vi "Simulator_Core.vi"(6 "NotifierReff":T1, 10 "disp_k":dbl=80.0, 11 "dt":dbl=1.0) -> ()   [LabVIEW 2013]
doc: "Simulator Core does a single time-step update (by dt), takes in only main position, jib position, and rudder position, and dt, (everything else is purely done by shift register and updates within the simulator), and outputs the new state variables and environmental conditions. Serves as the \"MODEL\" component of a model-view-controller simulation.\n\nSimulates based on ratios between expected behavior and modifying conditions rather than attempting and then kludging a force model. See the accompanying document for expanation of modeling decisions."
uses:
  cRIO_Code/Data/TypeDefs/Notifiers.ctl
  cRIO_Code/Data/TypeDefs/UTM Location.ctl
  cRIO_Code/Data/TypeDefs/Sail Set Suggestions.ctl
  cRIO_Code/Data/TypeDefs/Rudder Set Suggestions.ctl
  cRIO_Code/Data/TypeDefs/OverrideInformation.ctl
  cRIO_Code/Data/TypeDefs/OverrideMode.ctl
  cRIO_Code/Data/TypeDefs/MotorSetup.ctl
  cRIO_Code/Data/TypeDefs/DynamixelSetupInfo.ctl
  cRIO_Code/Data/TypeDefs/AirmarStatus.ctl
  cRIO_Code/Data/TypeDefs/HardwareOnline.ctl
  cRIO_Code/Data/TypeDefs/DynamixelCycleTracker.ctl
  cRIO_Code/Data/TypeDefs/RC Input Values.ctl
  cRIO_Code/Logic/Classes/Missions/GenericMission/GenericMission.lvclass
  cRIO_Code/Logic/Classes/Waypoint/Waypoint.lvclass
panel:
  out "rel_wind":dbl
  out "rel_wind_comp":dbl
  out "angular_drag":dbl
  out "Ts":dbl
  out "Tr":dbl
  out "RobotSp":dbl
  out "Vmax":dbl
  out "Vtmax":dbl
  out "SimLoopCounter":i32
  out "RelWindAngle":dbl
  out "JibP":dbl
  out "MainP":dbl
  out "WindSpeed":dbl
  out "AbsWindDirection":dbl(knob)
  out "RobotH":dbl(knob)
  out "PosY":dbl(graph)
  out "PosX":dbl(graph)
  out "VelY":dbl(graph)
  out "VelX":dbl(graph)
  out "Angular Velocity":dbl(graph)
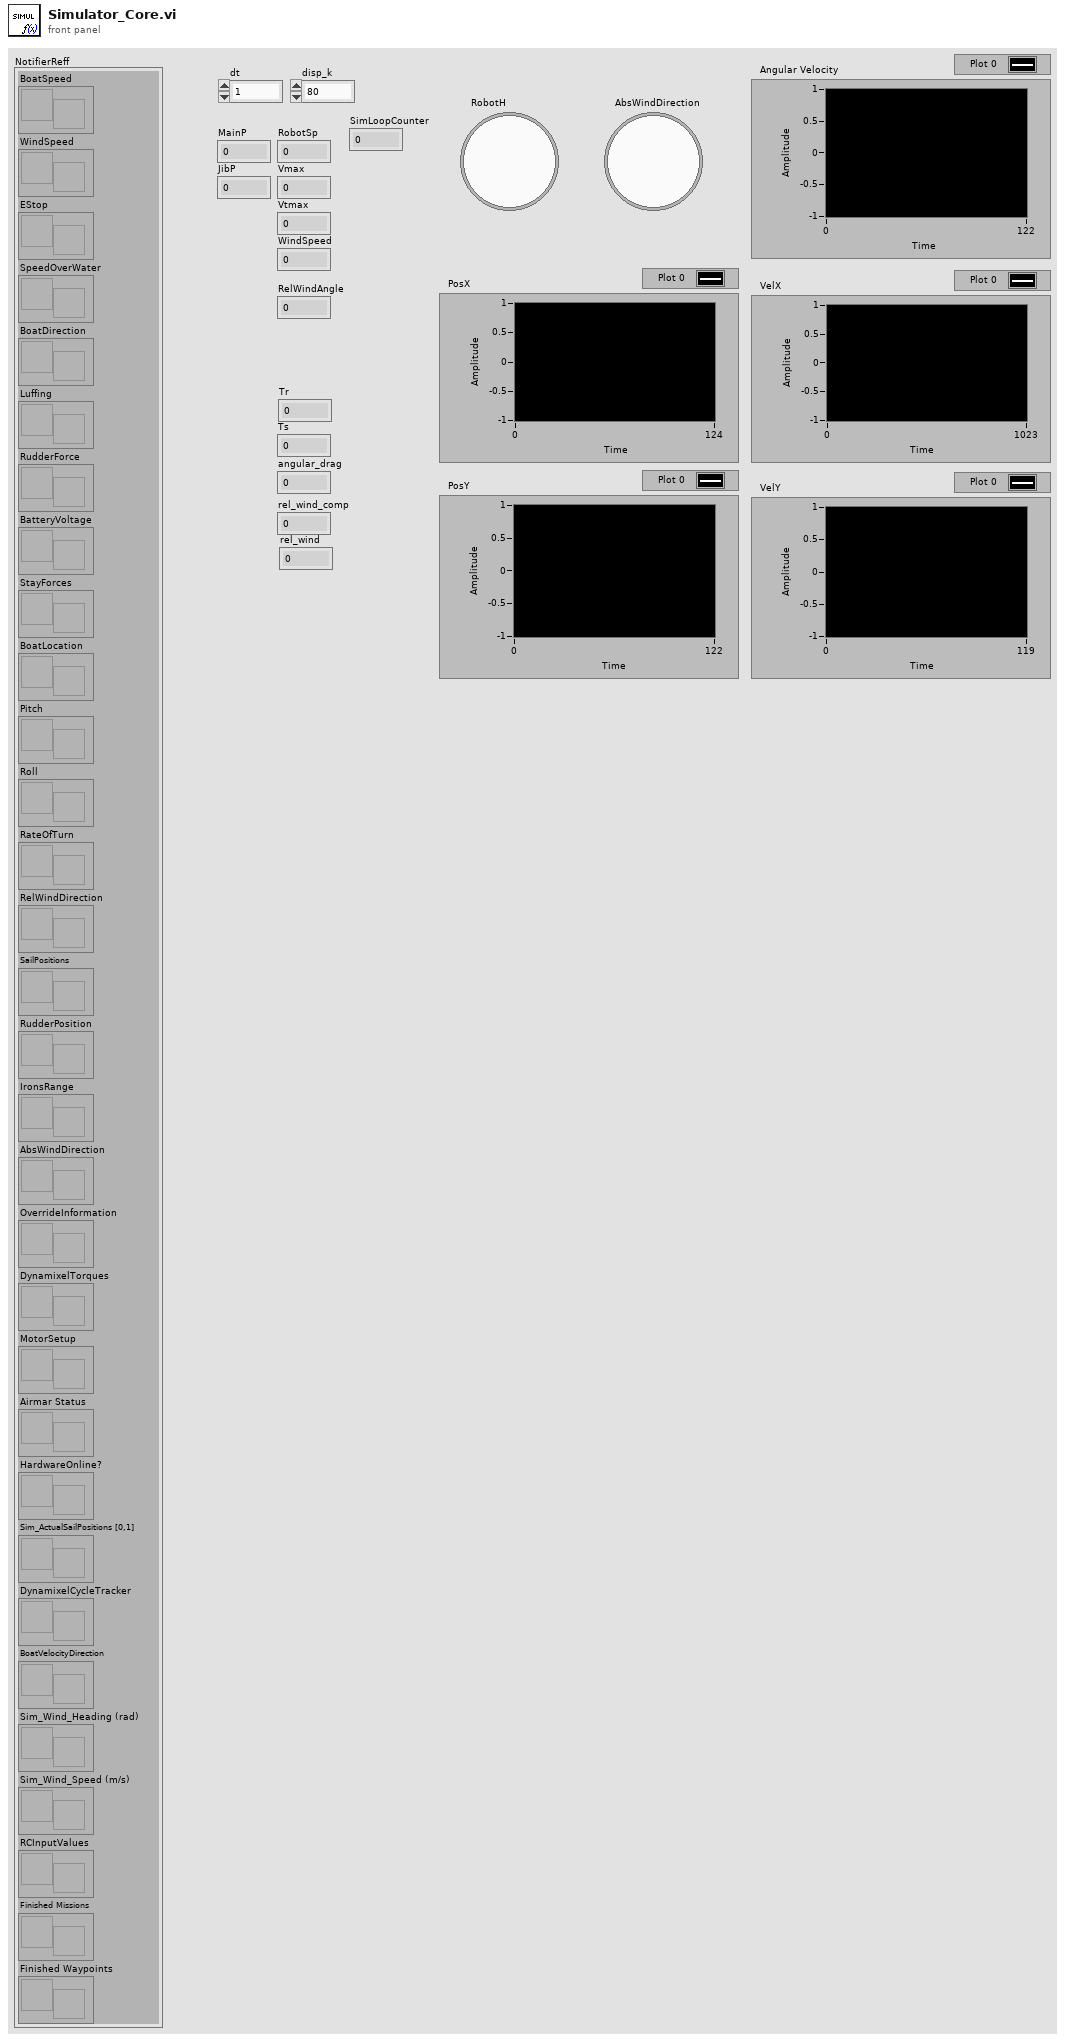
[diagram p1: front panel]
types:
  T1 = typedef "Notifiers.ctl" = cluster{"BoatSpeed":refnum<notifier>, "WindSpeed":refnum<notifier>, "EStop":refnum<notifier>, "SpeedOverWater":refnum<notifier>, "BoatDirection":refnum<notifier>, "Luffing":refnum<notifier>, "RudderForce":refnum<notifier>, "BatteryVoltage":refnum<notifier>, "StayForces":refnum<notifier>, "BoatLocation":refnum<notifier>, "Pitch":refnum<notifier>, "Roll":refnum<notifier>, "RateOfTurn":refnum<notifier>, "RelWindDirection":refnum<notifier>, "SailPositions":refnum<notifier>, "RudderPosition":refnum<notifier>, "IronsRange":refnum<notifier>, "AbsWindDirection":refnum<notifier>, "OverrideInformation":refnum<notifier>, "DynamixelTorques":refnum<notifier>, "MotorSetup":refnum<notifier>, "Airmar Status":refnum<notifier>, "HardwareOnline?":refnum<notifier>, "Sim_ActualSailPositions [0,1]":refnum<notifier>, "DynamixelCycleTracker":refnum<notifier>, "BoatVelocityDirection":refnum<notifier>, "Sim_Wind_Heading (rad)":refnum<notifier>, "Sim_Wind_Speed (m/s)":refnum<notifier>, "RCInputValues":refnum<notifier>, "Finished Missions":refnum<notifier>, "Finished Waypoints":refnum<notifier>}
  T2 = typedef "UTM Location.ctl" = cluster{"UTM Zone":dbl, "Hemisphere":enum16{"North", "South"}, "East":dbl, "North":dbl}
  T3 = typedef "Rudder Set Suggestions.ctl" = dbl
  T4 = typedef "Sail Set Suggestions.ctl" = cluster{"MainSailSuggestion":dbl, "JibSailSuggestion":dbl}
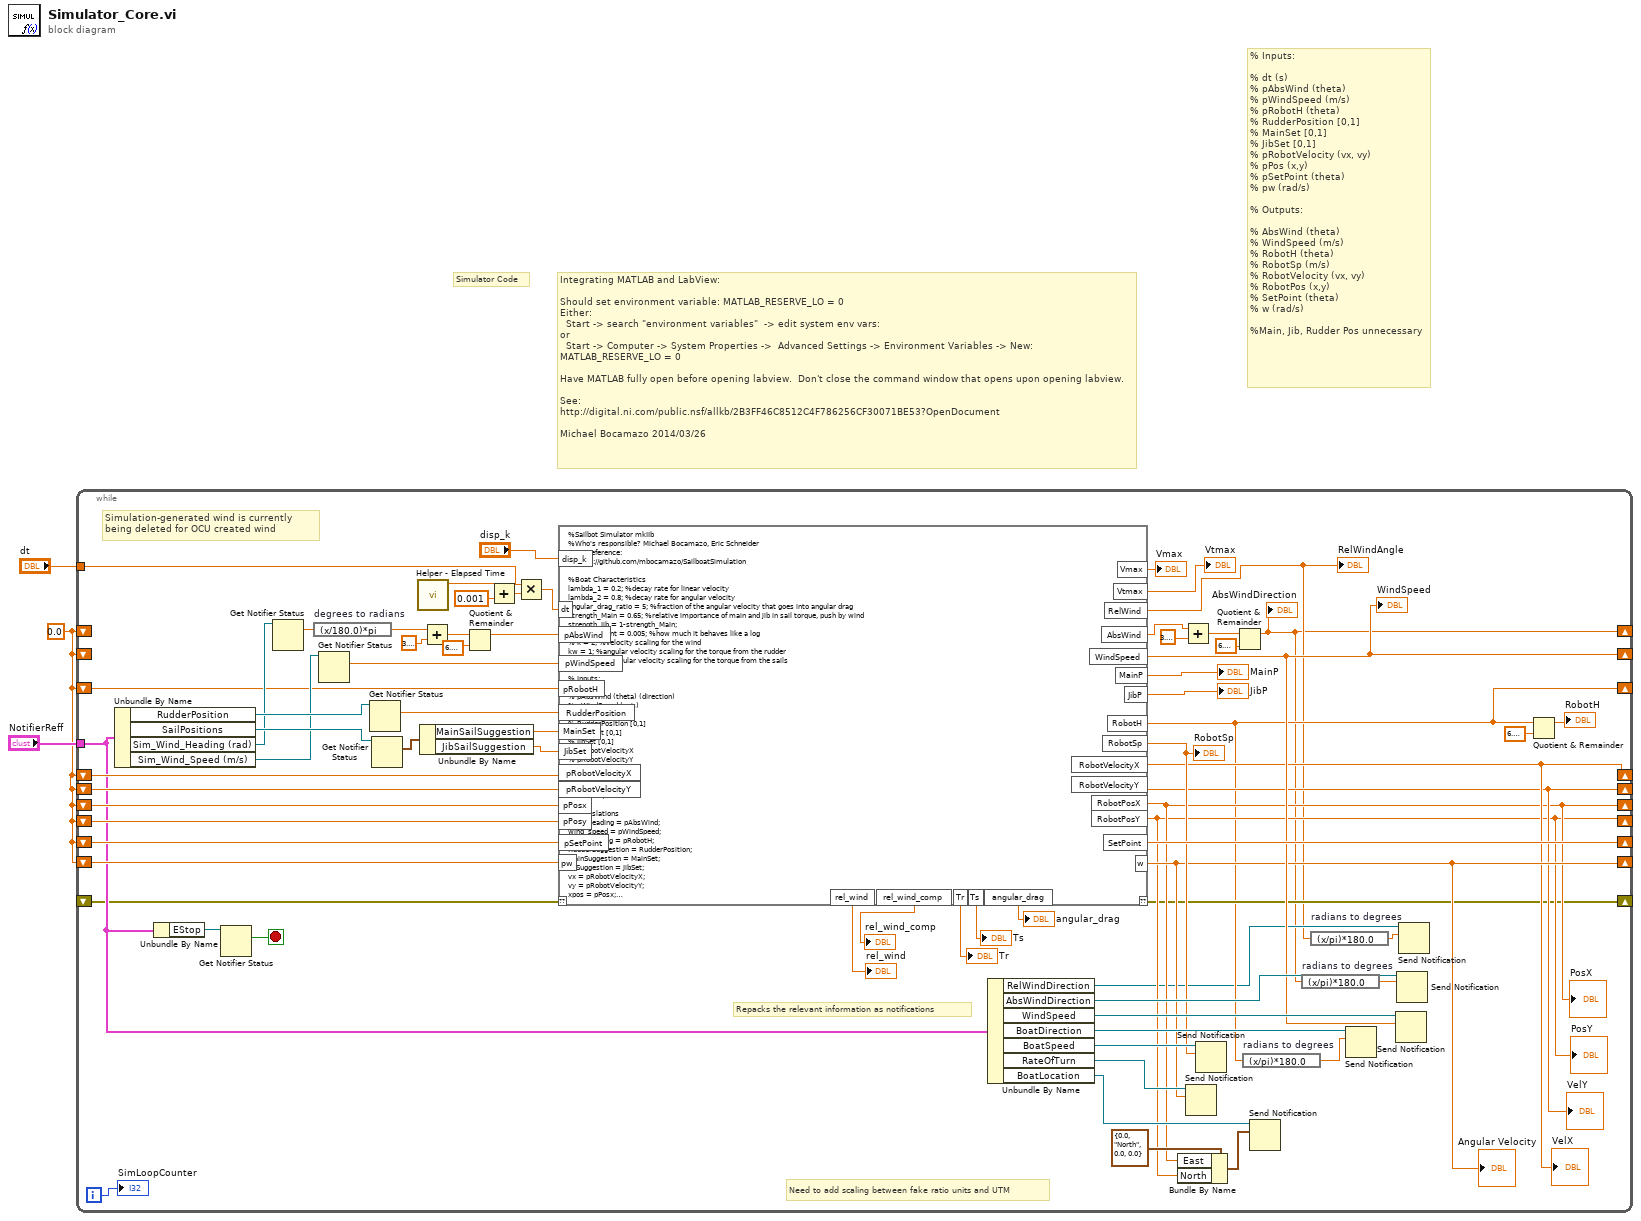
[diagram p0: block diagram]
diagram:
  w1 = 0.0
  # "% Inputs:\n\n% dt (s)\n% pAbsWind (theta)\n% pWindSpeed (m/s)\n% pRobotH (theta)\n% RudderPosition [0,1]\n% MainSet [0,1]\n% JibSet [0,1]\n% pRobotVelocity (vx, vy)\n% pPos (x,y)\n% pSetPoint (theta)\n% pw (rad/s)\n\n% Outputs:\n\n% AbsWind (theta)\n% WindSpeed (m/s)\n% RobotH (theta)\n% RobotSp (m/s)\n% RobotVelocity (vx, vy)\n% RobotPos (x,y)\n% SetPoint (theta)\n% w (rad/s)\n\n%Main, Jib, Rudder Pos unnecessary"
  # "Integrating MATLAB and LabView:\n\nShould set environment variable: MATLAB_RESERVE_LO = 0\nEither:\n  Start -> search \"environment variables\"  -> edit system env vars:\nor\n  Start -> Computer -> System Properties ->  Advanced Settings -> Environment Variables -> New:\nMATLAB_RESERVE_LO = 0 \n\nHave MATLAB fully open before opening labview.  Don't close the command window that opens upon opening labview.   \n\nSee:\nhttp://digital.ni.com/public.nsf/allkb/2B3FF46C8512C4F786256CF30071BE53?OpenDocument\n\nMichael Bocamazo 2014/03/26"
  # "Simulator Code"
  n1 = while {
    shift-right: [w54] -> _
    shift-left: w1 -> [w75]
    shift-right: [w74] -> _
    shift-left: w1 -> [w73]
    shift-right: [w51] -> _
    shift-left: w1 -> [w58]
    shift-right: [w12] -> _
    shift-left: w1 -> [_]
    shift-right: [w67] -> _
    shift-left: w1 -> [_]
    shift-right: [w33] -> _
    shift-left: w1 -> [w11]
    shift-right: [w52] -> _
    shift-left: w1 -> [w55]
    tunnel: "dt" -> [w10]
    tunnel: "NotifierReff" -> [w49]
    shift-right: [w50] -> _
    shift-left: w1 -> [w57]
    shift-right: [w53] -> _
    shift-left: w1 -> [w56]
    shift-right: [w44] -> _
    shift-left: _ -> [w43]
    i -> [w37]
    stop <- w47 stop-if-true
    # "Simulation-generated wind is currently being deleted for OCU created wind"
    # "Need to add scaling between fake ratio units and UTM"
    # "Repacks the relevant information as notifications"
    n2 = Unbundle By Name(w49) -> ("RudderPosition"=w72:refnum<notifier>, "SailPositions"=w70:refnum<notifier>, "Sim_Wind_Heading (rad)"=w31:refnum<notifier>, "Sim_Wind_Speed (m/s)"=w30:refnum<notifier>)
    n3 = Unbundle By Name(w49) -> ("EStop"=w48:refnum<notifier>)
    n4 = Get Notifier Status(notifier=w48) -> (current notification=w47:bool)  [unwired: 1 in, 4 out]
    n5 = Get Notifier Status(notifier=w31) -> (current notification=w23:dbl)  [unwired: 1 in, 4 out]
    n6 = expression code="(x/180.0)*pi" "degrees to radians"(w23) -> (w22:dbl)
    n7 = Get Notifier Status(notifier=w30) -> (current notification=w29:dbl)  [unwired: 1 in, 4 out]
    n8 = Get Notifier Status(notifier=w72) -> (current notification=w71:T3)  [unwired: 1 in, 4 out]
    n9 = Get Notifier Status(notifier=w70) -> (current notification=w59:T4)  [unwired: 1 in, 4 out]
    n10 = call "Helper - Elapsed Time.vi"() -> ("Time Elapsed (s)\nSince Last Iteration"=w28:dbl)  [unwired: 10 in, 1 out]
    n11 = Unbundle By Name(w59) -> ("MainSailSuggestion"=w46:dbl, "JibSailSuggestion"=w45:dbl)
    n12 = Add(x=w22, y=3.141592653589793) -> (x+y=w20:dbl)
    n13 = Quotient & Remainder(x=w20, y=6.283185307179586) -> (x-y*floor(x/y)=w18:dbl)  [unwired: 1 out]
    n14 = Add(x=w28, y=0.001) -> (x+y=w14:dbl)
    n15 = Multiply(x=w10, y=w14) -> (x*y=w13:dbl)
    n16 = script code="%Sailbot Simulator mkIIb\n%Who's responsible? Michael Bocamazo, Eric Schneider\n%For reference: \n%https://github.com/mbocamazo/SailboatSimulation\n\n%Boat Characteristics\nlambda_1 = 0.2; %decay rate for linear velocity\nlambda_2 = 0.8; %decay rate for angular velocity\nangular_drag_ratio = 5; %fraction of the angular velocity that goes into angular drag\nstrength_Main = 0.65; %relative importance of main and jib in sail torque, push by wind\nstrength_Jib = 1-strength_Main;\nlog_coefficient = 0.005; %how much it behaves like a log\n% k = 2; %velocity scaling for the wind\nkw = 1; %angular velocity scaling for the torque from the rudder\nks = 0.01; %angular velocity scaling for the torque from the sails\n\n% Inputs:\n% dt (s)\n% pAbsWind (theta) (direction)\n% pWindSpeed (m/s)\n% pRobotH (theta)\n% RudderPosition [0,1]\n% MainSet [0,1]\n% JibSet [0,1]\n% pRobotVelocityX\n% pRobotVelocityY\n% pPosx\n% pPosy\n% pSetPoint (theta)\n% pw (rad/s)\n\n% Translations\nwind_heading = pAbsWind;\nwind_speed = pWindSpeed;\nboat_heading = pRobotH;\nRudderSuggestion = RudderPosition;\nMainSuggestion = MainSet;\nJibSuggestion = JibSet;\nvx = pRobotVelocityX;\nvy = pRobotVelocityY;\nxpos = pPosx;\nypos = pPosy;\nangularVelocity = pw;\n\n\n% rel_wind is 0 when the wind is at the stern, and pi when the wind is blowing on the nose, even on both sides\nrel_wind = mod(abs(wind_heading-boat_heading),2*pi);\nif rel_wind > pi\n    % corrects to make the relative wind -pi to pi\n    rel_wind = 2.0*pi-rel_wind;\nend\n% rel_wind_comp is 0 when the wind is at the nose, and pi when the wind is blowing on the stern, even on both sides\nrel_wind_comp = pi-rel_wind;\n\n%Sanitization, possibly unnecessary\nwind_heading = mod(wind_heading,2*pi); \nboat_heading = mod(boat_heading,2*pi);\nif wind_speed <= 0\n    wind_speed = 0;\nend\n   \n%Trim based on what is possible\nRudderPos = RudderSuggestion;\nMainPos = min([MainSuggestion,rel_wind_comp*2.0/pi,1]); %in foolish ratio units, [0 1], 1 being full out, 90 degrees\nJibPos = min([JibSuggestion,rel_wind_comp*2.0/pi,1]);\nif mod(wind_heading-boat_heading,2*pi)<pi\n    wind_over_port = 1;\nelse\n    wind_over_port = 0;\nend\n\n%Calculate the forward speed\ndirection = atan2(vy,vx);\nspeed = norm([vx,vy]);\nforward_speed = cos(direction-boat_heading)*speed;\n\n%rudder torque aspect\n%the linear relationship means a faster boat speed results in a greater rudder effect\n%the negative sign is b/c a -1 rudder value (turn to port) results in a positive angular change (CCW)\nTr =  -kw*forward_speed*RudderPos;\n\nif wind_over_port  %non-intuitive reversal needs to be explained\n    reverse = -1;\nelse\n    reverse = 1;\nend\n    \n%ANGLES! Gets the absolute sail angles (relative to the world, not the boat)\nmain_angle = atan2(-sin(boat_heading+MainPos*pi/2.0*reverse),-cos(boat_heading+MainPos*pi/2.0*reverse));\njib_angle = atan2(-sin(boat_heading+JibPos*pi/2.0*reverse),-cos(boat_heading+JibPos*pi/2.0*reverse));\n\n%sail torque aspect\nTs = -ks*strength_Main*sin(main_angle-wind_heading)*sqrt(wind_speed); \nTs = Ts + ks*strength_Jib*sin(jib_angle-wind_heading)*sqrt(wind_speed); %Definitely Wrong, need to fix\n\n%effectively drag - the resistance to turning in a boat gets much higher when the boat is going faster\nangular_drag = -sign(angularVelocity)*angularVelocity^2*angular_drag_ratio;\nif isnan(angular_drag)\n    angularVelocity = 0;\nelse\n    angularVelocity = angularVelocity + lambda_2*(angular_drag+Tr+Ts)*dt;\n    % angularVelocity = angularVelocity + lambda_2*(angular_drag+Tr)*dt;\n    % angularVelocity = angularVelocity + lambda_2*(Tr)*dt;\nend\n\n%forward sail aspect\nif rel_wind_comp > pi/2\n    Sr = 0;\nelse\n    Sr = 2/pi*rel_wind_comp-1;\nend\n\n% the 0.0001 factor is to prevent divide by 0 error\nPrMain = sin(pi^2/(4*rel_wind_comp + 0.0001)*MainPos)*strength_Main;\nPrJib = sin(pi^2/(4*rel_wind_comp + 0.0001)*JibPos)*strength_Jib;\n\nDr = 1-0.9*sin(abs(RudderPos*pi/2));\n\n% ratios a, b, c made up\npiece1_root1 = -0.78\npiece1_root2 = 0.78\npiece1_scaling = 0.05\npiece2_root1 = -3 - 1.57\npiece2_root2 = 3 - 1.57\npiece2_scaling = -0.11\n\nif (rel_wind_comp < pi/4)\n    Vtmax = wind_speed*piece1_scaling*(rel_wind_comp + piece1_root1)*(rel_wind_comp + piece1_root2)\nelse\n    Vtmax = wind_speed*piece2_scaling*(rel_wind_comp + piece2_root1)*(rel_wind_comp + piece2_root2)\nend\nVmax = Vtmax*(PrMain+(1-Sr)*PrJib)/(2.0-Sr)*Dr;\nforward_speed = forward_speed + lambda_1*(Vmax-forward_speed)*dt; %decay to the max, acceleration term\n\n%conversion to cartesian\nvx = forward_speed*cos(boat_heading);\nvy = forward_speed*sin(boat_heading);\n\n% floating log aspect (in cartesian, rather than doing vector addition, which is also possible)    \nvx = vx + wind_speed*cos(wind_heading)*log_coefficient*dt;\nvy = vy + wind_speed*sin(wind_heading)*log_coefficient*dt;\n\n%finally, updates\nboat_heading = boat_heading + angularVelocity*dt;\nxpos = xpos + vx*dt*disp_k;\nypos = ypos + vy*dt*disp_k;\n\n% Outputs:\nRelWind = rel_wind_comp;\nAbsWind = wind_heading;\nSetPoint = wind_heading; %different if programmed wind change\nWindSpeed = wind_speed;\nMainP = MainPos;\nJibP = JibPos;\nRobotH = boat_heading;\nRobotSp = forward_speed; %unresolved question of perpendicular velocity\n\nRobotVelocityX = vx;\nRobotVelocityY = vy;\nRobotPosX = xpos;\nRobotPosY = ypos;\nw = angularVelocity;\n\n%     xpos = xpos\n%     ypos = ypos\n%     MainPos = 0\n%     JibPos = 0\n%     MainSuggestion = 0\n%     JibSuggestion = 0\n%     RudderPos = 0\n%     RudderSuggestion = 0\n%     vx = 0\n%     vy = 0\n%     heading = 0 %note: not redundant with vx, vy; in simple model could be\n%     angularVelocity = 0\n%     forward_speed = 0\n%     wind_over_port = True \n%     log_coefficient = 0.1\n%     lambda_1 = 0.1 %can't be named lambda, reserved\n%     lambda_2 = 0.4 %decay rate for angular velocity, to zero, way of encoding drag\n%     strength_Main = 0.65\n%     strength_Jib = 1-strength_Main\n%     main_angle = 0\n%     jib_angle = 0"("??"=w43, "dt"=w13, "pAbsWind"=w18, "pWindSpeed"=w29, "pRobotH"=w11, "RudderPosition"=w71, "MainSet"=w46, "JibSet"=w45, "pRobotVelocityX"=w56, "pPosx"=w58, "pSetPoint"=w73, "pw"=w75, "pPosy"=w57, "pRobotVelocityY"=w55, "disp_k"="disp_k") -> ("??"=w44:errorcluster, "SetPoint"=w74:dbl, "AbsWind"=w16:dbl, "WindSpeed"=w67:dbl, "RobotSp"=w64:dbl, "RobotVelocityX"=w53:dbl, "RobotPosX"=w51:dbl, "RobotH"=w33:dbl, "w"=w54:dbl, "RobotPosY"=w50:dbl, "RobotVelocityY"=w52:dbl, "RelWind"=w24:dbl, "MainP"=→"MainP":dbl, "JibP"=→"JibP":dbl, "Vtmax"=→"Vtmax":dbl, "Vmax"=→"Vmax":dbl, "Tr"=→"Tr":dbl, "Ts"=→"Ts":dbl, "angular_drag"=→"angular_drag":dbl, "rel_wind_comp"=→"rel_wind_comp":dbl, "rel_wind"=→"rel_wind":dbl)
    "Angular Velocity" <- w54
    "VelX" <- w53
    "VelY" <- w52
    "PosX" <- w51
    "PosY" <- w50
    "WindSpeed" <- w67
    "RelWindAngle" <- w24
    "RobotSp" <- w64
    n17 = Unbundle By Name(w49) -> ("RelWindDirection"=w26:refnum<notifier>, "AbsWindDirection"=w69:refnum<notifier>, "WindSpeed"=w68:refnum<notifier>, "BoatDirection"=w66:refnum<notifier>, "BoatSpeed"=w65:refnum<notifier>, "RateOfTurn"=w63:refnum<notifier>, "BoatLocation"=w62:refnum<notifier>)
    n18 = Bundle By Name(cluster=T2 {"UTM Zone"=0.0, "Hemisphere"=enum."North", "East"=0.0, "North"=0.0} ("UTM Location"), "East"=w51, "North"=w50) -> (w60:T2)
    n19 = Add(x=w16, y=3.141592653589793) -> (x+y=w15:dbl)
    n20 = Send Notification(notification=w54, notifier=w63) -> ()  [unwired: 1 in, 2 out]
    n21 = Send Notification(notification=w64, notifier=w65) -> ()  [unwired: 1 in, 2 out]
    n22 = Quotient & Remainder(x=w15, y=6.283185307179586) -> (x-y*floor(x/y)=w12:dbl)  [unwired: 1 out]
    "AbsWindDirection" <- w12
    n23 = expression code="(x/pi)*180.0" "radians to degrees"(w33) -> (w32:dbl)
    n24 = Send Notification(notification=w60, notifier=w62) -> ()  [unwired: 1 in, 2 out]
    n25 = expression code="(x/pi)*180.0" "radians to degrees"(w12) -> (w34:dbl)
    n26 = expression code="(x/pi)*180.0" "radians to degrees"(w24) -> (w25:dbl)
    n27 = Send Notification(notification=w32, notifier=w66) -> ()  [unwired: 1 in, 2 out]
    n28 = Send Notification(notification=w67, notifier=w68) -> ()  [unwired: 1 in, 2 out]
    n29 = Send Notification(notification=w34, notifier=w69) -> ()  [unwired: 1 in, 2 out]
    n30 = Send Notification(notification=w25, notifier=w26) -> ()  [unwired: 1 in, 2 out]
    n31 = Quotient & Remainder(x=w33, y=6.283185307179586) -> (x-y*floor(x/y)=→"RobotH":dbl)  [unwired: 1 out]
    "SimLoopCounter" <- w37
  }
